vi "Display Info.vi"(7 "Layout ref":refnum<vi>, 8 "error in (no error)":errorcluster, 9 "Modify (F) /Add [T]":bool=TRUE, 10 "Names in use":string[](array[string])=["PulseBlaster", "NI card_0", "NI card_1", "NI card_2", "NI card_3", "SRS_0", "RedDDSArd", "BlueBNArd", "PIXIS_Linear_Act"], 11 "DMD in":refnum<class "DMD.lvclass">=refnum) -> (0 "error out":errorcluster, 1 "Names in use out":string[](array[string]), 2 "Changes Made?":bool, 3 "DMD out":refnum<class "DMD.lvclass">)   [LabVIEW 2013, in "DMD.lvclass"]
uses:
  DMD.lvclass
  ColumnVIs/SingleValCol/SingleValCol.lvclass
  ColumnVIs/SingleValMenuCol/SingleValMenuCol.lvclass
  TypeDefs/ColumnAppearCluster.ctl
  DMD.lvclass/DMD.ctl
  ColumnVIs/Column/Column.lvclass
panel:
  in  "Program Mode Appearance":T1={"Column Name"="Program Mode", "Width"=30, "Bkgd"=[16448250], "Text"=[0]}
  in  "Display Mode Appearance":T1={"Column Name"="Disp Mode", "Width"=30, "Bkgd"=[16448250], "Text"=[0]}
  in  "Pattern Name Appearance":T1={"Column Name"="Pattern Name", "Width"=30, "Bkgd"=[16448250], "Text"=[0]}
  in  "Imgs in Pattern Appearance":T1={"Column Name"="Num Images", "Width"=30, "Bkgd"=[16448250], "Text"=[0]}
  in  "Device Description":string
  in  "Hardware Settings":T2 {"Port" format="%x"}
  in  "Name":string
  in  "Done":bool
  in  "Cancel":bool
  # "Always use Port 0x5555\nPort Field is in Hexadecimal"
  # "Use IP addresses in: \n172.16.0.0 to 172.16.255.255\nor\n192.168.0.0 to 192.168.255.255\n\nNote: Most DMDs default to\n192.168.1.100\n\nIf another IP is needed it must be \nset with the DMD software."
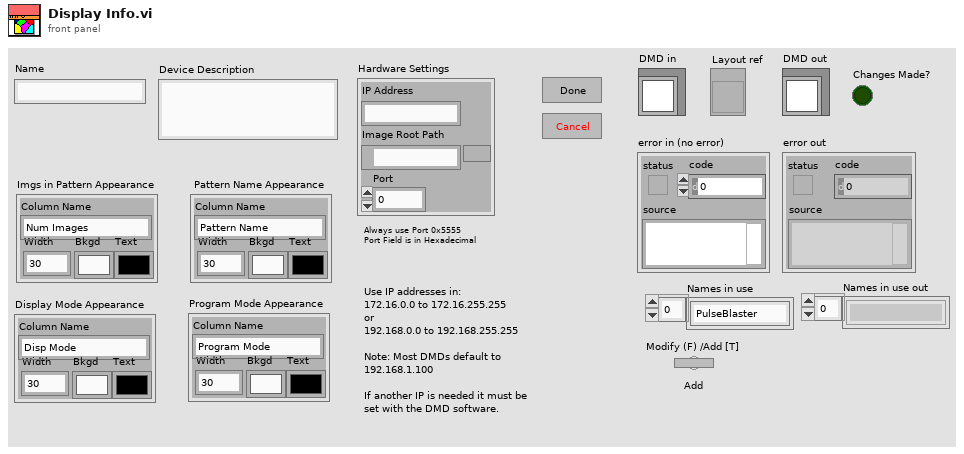
[diagram p1: front panel]
types:
  T1 = typedef "ColumnAppearCluster.ctl" = cluster{"Column Name":string, "Width":u32, "Bkgd":u32[], "Text":u32[]}
  T2 = cluster{"IP Address":string, "Image Root Path":path, "Port":u16}
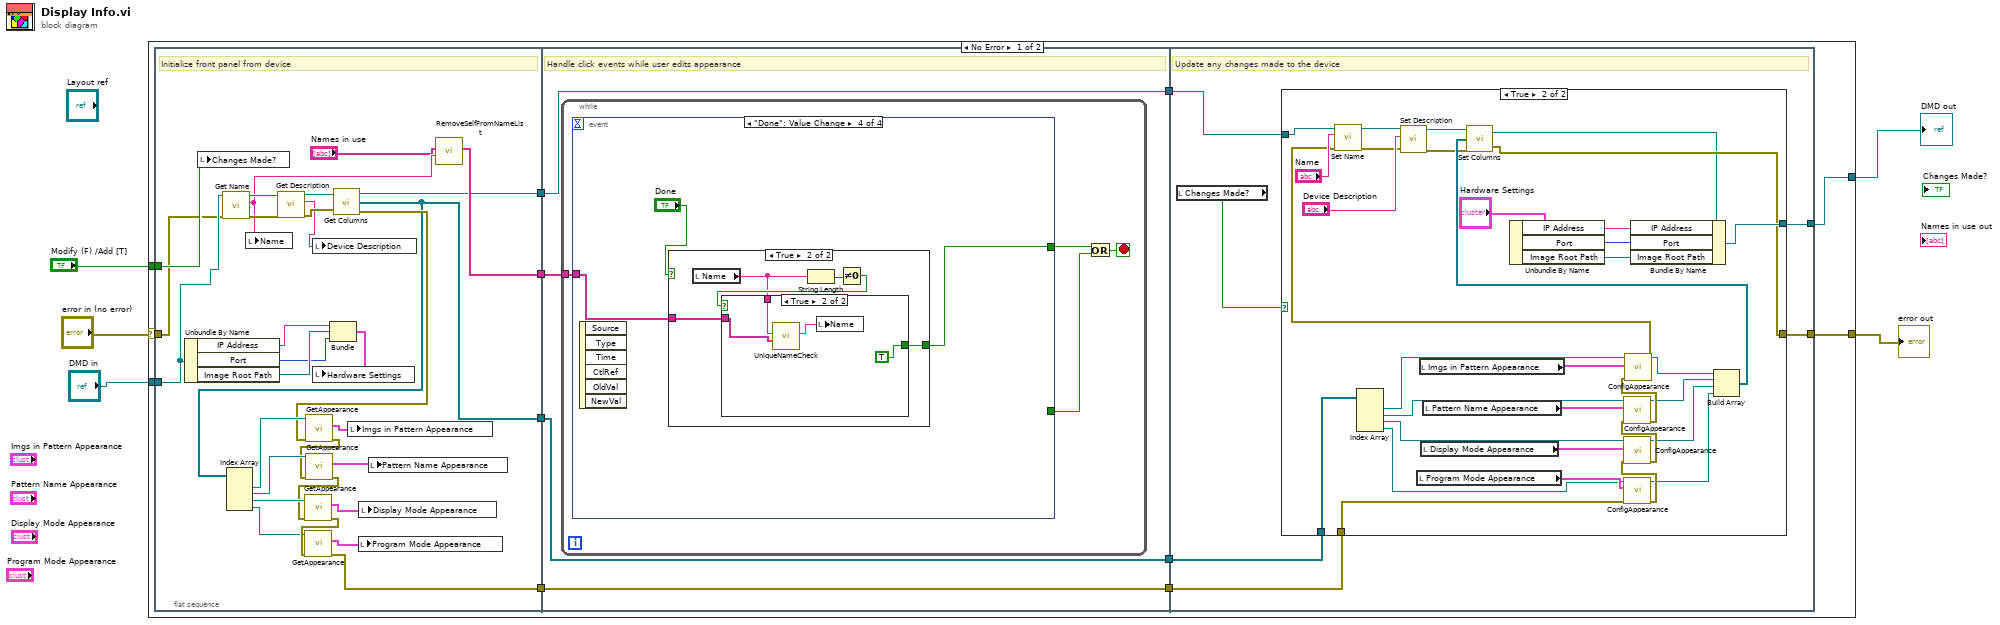
[diagram p0: block diagram]
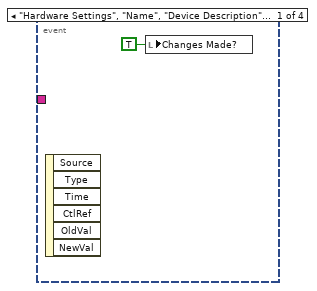
[diagram p2: hidden frame]
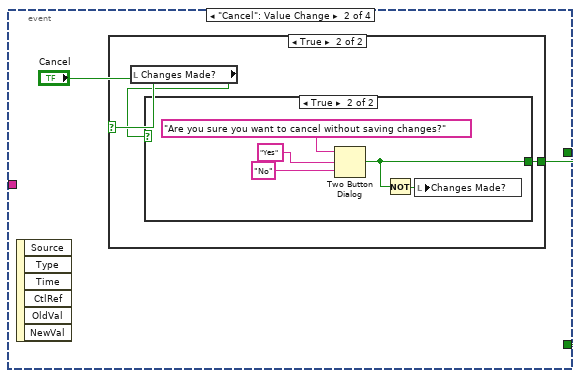
[diagram p3: hidden frame]
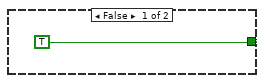
[diagram p5: hidden frame]
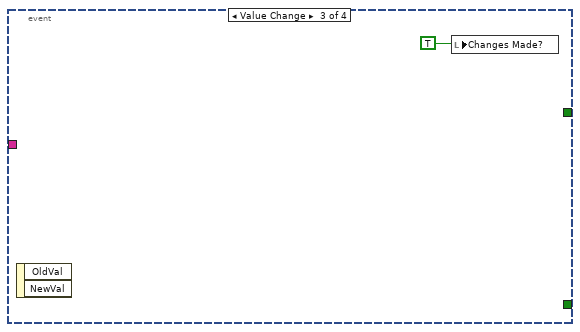
[diagram p6: hidden frame]
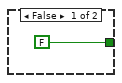
[diagram p7: hidden frame]
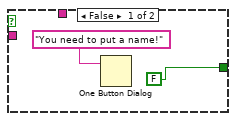
[diagram p8: hidden frame]
diagram:
  n1 = case shown="No Error" "error in (no error)" {
    selector: "error in (no error)" -> [w15 w126]
    tunnel: [w7 w126] -> w1
    tunnel: [w6 w125] -> w2
    tunnel: "DMD in" -> [w16 w125]
    tunnel: "Modify (F) /Add [T]" -> [w17 _]
    frame No Error {
      n2 = flat-sequence {
        tunnel: w17 -> [w47]
        tunnel: w16 -> [w45]
        tunnel: w15 -> [w43]
        tunnel: [w28] -> w14
        tunnel: [w27] -> w13
        tunnel: [w26] -> w11
        tunnel: [w20] -> w9
        tunnel: w14 -> [w51]
        tunnel: w13 -> [w50]
        tunnel: [w50] -> w12
        tunnel: w11 -> [w49]
        tunnel: [w49] -> w10
        tunnel: w9 -> [w48]
        tunnel: [w48] -> w8
        tunnel: w12 -> [w89]
        tunnel: w10 -> [w88]
        tunnel: w8 -> [w87]
        tunnel: [w85] -> w7
        tunnel: [w84] -> w6
        frame #0 {
          # "Initialize front panel from device"
          n3 = Unbundle By Name(w45) -> ("IP Address"=w46:string, "Port"=w23:u16, "Image Root Path"=w24:path)
          n4 = local write "Changes Made?"(w47) -> ()
          n5 = call-dynamic "Get Name.vi"("error in (no error)"=w43, "Device in"=w45) -> ("error out"=w42:errorcluster, "Name"=w39:string, "Device out"=w44:refnum<class "DMD.lvclass">)  [unwired: 7 in]
          n6 = local write "Name"(w39) -> ()
          n7 = call-dynamic "Get Description.vi"("error in (no error)"=w42, "Device in"=w44) -> ("error out"=w40:errorcluster, "Device Description"=w38:string, "Device out"=w41:refnum<class "DMD.lvclass">)  [unwired: 7 in]
          n8 = local write "Device Description"(w38) -> ()
          n9 = Bundle("IP Address"=w46, "Image Root Path"=w24, "Port"=w23) -> (w22:T2)  [unwired: 1 in]
          n10 = local write "Hardware Settings"(w22) -> ()
          n11 = call-dynamic "Get Columns.vi"("Device in"=w41, "error in (no error)"=w40) -> ("Device out"=w27:refnum<class "DMD.lvclass">, "Columns"=w26:refnum<class "Column.lvclass">[], "error out"=w34:errorcluster)
          n12 = Index Array(array=w26) -> (element #1=w37:refnum<class "Column.lvclass">, element #2=w36:refnum<class "Column.lvclass">, element #3=w35:refnum<class "Column.lvclass">, element #4=w19:refnum<class "Column.lvclass">)  [unwired: 4 in]
          n13 = call "GetAppearance.vi"("error in (no error)"=w34, "Column in"=w37) -> ("error out"=w33:errorcluster, "Column Appearance"=w31:T1)  [unwired: 7 in, 1 out]
          n14 = call "GetAppearance.vi"("error in (no error)"=w33, "Column in"=w36) -> ("error out"=w32:errorcluster, "Column Appearance"=w30:T1)  [unwired: 7 in, 1 out]
          n15 = call "GetAppearance.vi"("error in (no error)"=w32, "Column in"=w35) -> ("error out"=w21:errorcluster, "Column Appearance"=w29:T1)  [unwired: 7 in, 1 out]
          n16 = call "GetAppearance.vi"("error in (no error)"=w21, "Column in"=w19) -> ("error out"=w20:errorcluster, "Column Appearance"=w18:T1)  [unwired: 7 in, 1 out]
          n17 = local write "Imgs in Pattern Appearance"(w31) -> ()
          n18 = local write "Program Mode Appearance"(w18) -> ()
          n19 = local write "Display Mode Appearance"(w29) -> ()
          n20 = local write "Pattern Name Appearance"(w30) -> ()
          n21 = call "RemoveSelfFromNameList.vi"("self Name"=w39, "Names in use"="Names in use") -> ("Reserved Names"=w28:string[])  [unwired: 9 in]
        }
        frame #1 {
          # "Handle click events while user edits appearance"
          n22 = while {
            tunnel: w51 -> [w52]
            stop <- w55 stop-if-true
            n23 = event shown="[3] \"Done\": Value Change" {
              selector: _ -> [_ _ _ _]
              dyn-events: _ -> [_ _ _ _]
              timeout: _ -> [_ _ _ _]
              tunnel: [_ w58 _ _] -> w54
              tunnel: [_ _ _ w71] -> w53
              tunnel: w52 -> [_ _ _ w69]
              event "Hardware Settings", "Name", "Device Description": Value Change {
                n24 = event-data() -> ()  [unwired: 1 in, 6 out]
                n25 = local write "Changes Made?"(TRUE ("Changes Made?")) -> ()
              }
              event "Cancel": Value Change {
                n26 = event-data() -> ()  [unwired: 1 in, 6 out]
                n27 = case shown="True" "Cancel" {
                  selector: "Cancel" -> [w59 _]
                  tunnel: [w59 w61] -> w58
                  frame False {
                  }
                  frame True {
                    n28 = local read "Changes Made?"() -> (w60:bool)
                    n29 = case shown="True" w60 {
                      tunnel: [TRUE w64] -> w61
                      frame False {
                      }
                      frame True {
                        n30 = Two Button Dialog(message="Are you sure you want to cancel without saving changes?", 1:"No", 2:"Yes") -> (T button?=w64:bool)
                        n31 = Not(x=w64) -> (.not. x?=w63:bool)
                        n32 = local write "Changes Made?"(w63) -> ()
                      }
                    }
                  }
                }
              }
              event Value Change {
                n33 = event-data() -> ()  [unwired: 1 in, 2 out]
                n34 = local write "Changes Made?"(TRUE) -> ()
              }
              event "Done": Value Change {
                n35 = event-data() -> ()  [unwired: 1 in, 6 out]
                n36 = case shown="True" "Done" {
                  tunnel: [FALSE w75] -> w71
                  tunnel: w69 -> [_ w74]
                  frame False {
                  }
                  frame True {
                    n37 = local read "Name"() -> (w73:string)
                    n38 = String Length(string=w73) -> (length=w77:i32)
                    n39 = Not Equal To 0?(x=w77) -> (x != 0?=w76:bool)
                    n40 = case shown="True" w76 {
                      tunnel: [FALSE TRUE] -> w75
                      tunnel: w74 -> [_ w82]
                      tunnel: w73 -> [_ w81]
                      frame False {
                        n41 = One Button Dialog(message="You need to put a name!") -> ()  [unwired: 1 in, 1 out]
                      }
                      frame True {
                        n42 = call "UniqueNameCheck.vi"("Names in use"=w82, "Device Name"=w81) -> ("Unique name"=w80:string)  [unwired: 8 in, 1 out]
                        n43 = local write "Name"(w80) -> ()
                      }
                    }
                  }
                }
              }
            }
            n44 = Or(x=w53, y=w54) -> (x .or. y?=w55:bool)
          }
        }
        frame #2 {
          # "Update any changes made to the device"
          n45 = local read "Changes Made?"() -> (w86:bool)
          n46 = case shown="True" w86 {
            tunnel: w89 -> [w91 w124]
            tunnel: w88 -> [_ w119]
            tunnel: w87 -> [w90 w96]
            tunnel: [w90 w98] -> w85
            tunnel: [w91 w101] -> w84
            frame False {
            }
            frame True {
              n47 = Index Array(array=w119) -> (element #1=w118:refnum<class "Column.lvclass">, element #2=w117:refnum<class "Column.lvclass">, element #3=w116:refnum<class "Column.lvclass">, element #4=w93:refnum<class "Column.lvclass">)  [unwired: 4 in]
              n48 = local read "Program Mode Appearance"() -> (w94:T1)
              n49 = local read "Imgs in Pattern Appearance"() -> (w111:T1)
              n50 = local read "Display Mode Appearance"() -> (w109:T1)
              n51 = local read "Pattern Name Appearance"() -> (w110:T1)
              n52 = Unbundle By Name("Hardware Settings") -> ("IP Address"=w102:string, "Port"=w100:u16, "Image Root Path"=w99:path)
              n53 = call "ConfigAppearance.vi"("error in (no error)"=w96, "Column Appearance"=w94, "Column in"=w93) -> ("error out"=w95:errorcluster, "Column out"=w92:refnum<class "Column.lvclass">)  [unwired: 7 in]
              n54 = call "ConfigAppearance.vi"("error in (no error)"=w95, "Column Appearance"=w109, "Column in"=w116) -> ("error out"=w115:errorcluster, "Column out"=w106:refnum<class "Column.lvclass">)  [unwired: 7 in]
              n55 = call "ConfigAppearance.vi"("error in (no error)"=w115, "Column Appearance"=w110, "Column in"=w117) -> ("error out"=w114:errorcluster, "Column out"=w107:refnum<class "Column.lvclass">)  [unwired: 7 in]
              n56 = call "ConfigAppearance.vi"("error in (no error)"=w114, "Column Appearance"=w111, "Column in"=w118) -> ("error out"=w113:errorcluster, "Column out"=w108:refnum<class "Column.lvclass">)  [unwired: 7 in]
              n57 = call-dynamic "Set Name.vi"("error in (no error)"=w113, "Name"="Name", "Device in"=w124) -> ("error out"=w112:errorcluster, "Device out"=w122:refnum<class "DMD.lvclass">)  [unwired: 7 in]
              n58 = call-dynamic "Set Description.vi"("error in (no error)"=w112, "Device Description"="Device Description", "Device in"=w122) -> ("error out"=w103:errorcluster, "Device out"=w104:refnum<class "DMD.lvclass">)  [unwired: 7 in]
              n59 = Build Array(w108, w107, w106, w92) -> (w105:refnum<class "Column.lvclass">[])
              n60 = call-dynamic "Set Columns.vi"("error in (no error)"=w103, "Columns"=w105, "Device in"=w104) -> ("error out"=w98:errorcluster, "Device out"=w97:refnum<class "DMD.lvclass">)  [unwired: 1 in]
              n61 = Bundle By Name(cluster=w97, "IP Address"=w102, "Port"=w100, "Image Root Path"=w99) -> (w101:refnum<class "DMD.lvclass">)
            }
          }
        }
      }
    }
    frame Error {
    }
  }
  "error out" <- w1
  "DMD out" <- w2
